vi "Child_2 - SET -  Actor_Name.vi"(8 "error in (no error)":errorcluster, 10 "Actor_Name":string, 11 "Child_2_Class in":refnum<class "Child_2_Class.lvclass">=refnum) -> (0 "error out":errorcluster, 2 "Actor Name":string, 3 "Child_2_Class out":refnum<class "Child_2_Class.lvclass">)   [LabVIEW 2023, in "Actor_Child_2.lvlib" / "Child_2_Class.lvclass"]
uses:
  Child_2_Class.lvclass
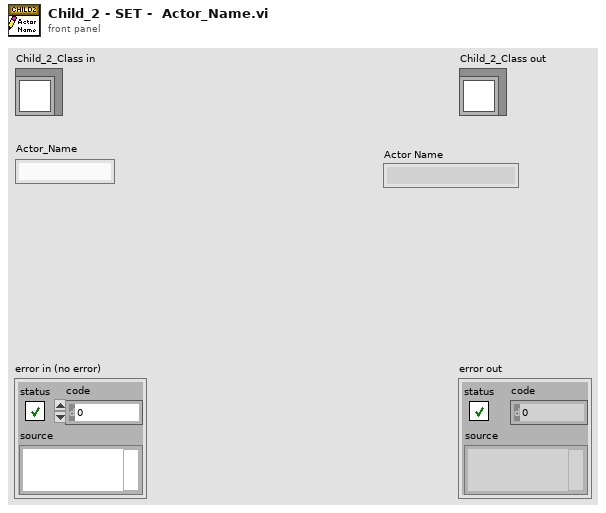
[diagram p1: front panel]
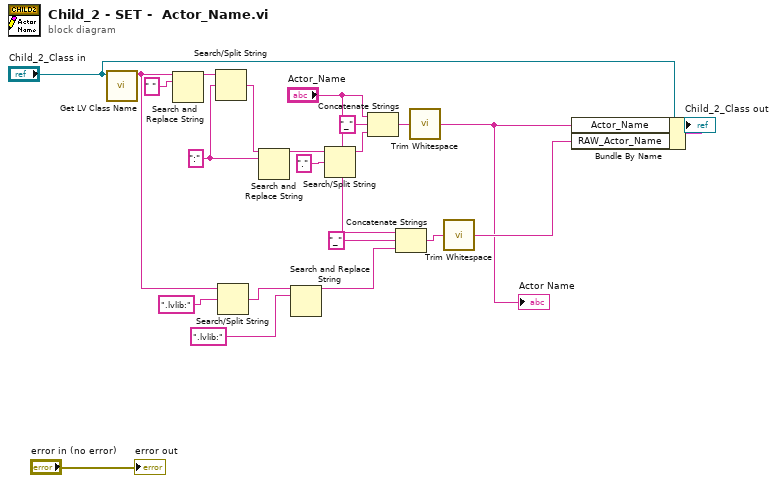
[diagram p0: block diagram]
diagram:
  w18 = ":" ("search string/char (-)")
  n1 = call <vilib>:"Get LV Class Name.vi"("object"="Child_2_Class in") -> ("class name"=w6:string)  [unwired: 9 in, 1 out]
  n2 = Search and Replace String(input string=w6, search string=" ") -> (result string=w20:string)  [unwired: 6 in, 3 out]
  n3 = Search/Split String(string=w20, search string/char (-)=w18) -> (match + rest of string=w19:string)  [unwired: 1 in, 2 out]
  n4 = Search/Split String(string=w6, search string/char (-)=".lvlib:") -> (match + rest of string=w9:string)  [unwired: 1 in, 2 out]
  n5 = Search and Replace String(input string=w19, search string=w18) -> (result string=w15:string)  [unwired: 6 in, 3 out]
  n6 = Search and Replace String(input string=w9, search string=".lvlib:" ("search string/char (-)")) -> (result string=w8:string)  [unwired: 6 in, 3 out]
  n7 = Search/Split String(string=w15, search string/char (-)=".") -> (substring before match=w13:string)  [unwired: 1 in, 2 out]
  n8 = Concatenate Strings("Actor_Name", "_" ("string"), w13) -> (w16:string)
  n9 = Concatenate Strings("Actor_Name", "_" ("string"), w8) -> (w7:string)
  n10 = call <vilib>:"Trim Whitespace.vi"("string"=w16) -> ("trimmed string"=w4:string)  [unwired: 1 in]
  "Actor Name" <- w4
  n11 = call <vilib>:"Trim Whitespace.vi"("string"=w7) -> ("trimmed string"=w5:string)  [unwired: 1 in]
  n12 = Bundle By Name(cluster="Child_2_Class in", "Actor_Name"=w4, "RAW_Actor_Name"=w5) -> (→"Child_2_Class out":cluster{})
  "error out" <- "error in (no error)"
